vi "Set and get merit factor array.vi"(7 "action":enum16{"set", "get", "initialise"}(ring)=enum."initialise", 8 "error in (no error)":errorcluster, 9 "array size":i32=5, 10 "merit factor":dbl, 11 "RSA in":refnum<class "RSA.lvclass">) -> (0 "error out":errorcluster, 1 "current merit factor":dbl, 2 "merit factor array":dbl[](array[numeric]), 3 "RSA out":refnum<class "RSA.lvclass">)   [LabVIEW 2012, in "RSA.lvclass"]
uses:
  RSA.lvclass
  RSA.lvclass/RSA.ctl
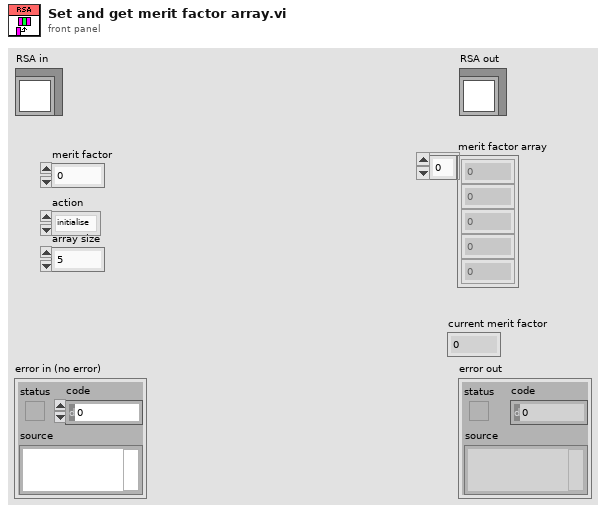
[diagram p1: front panel]
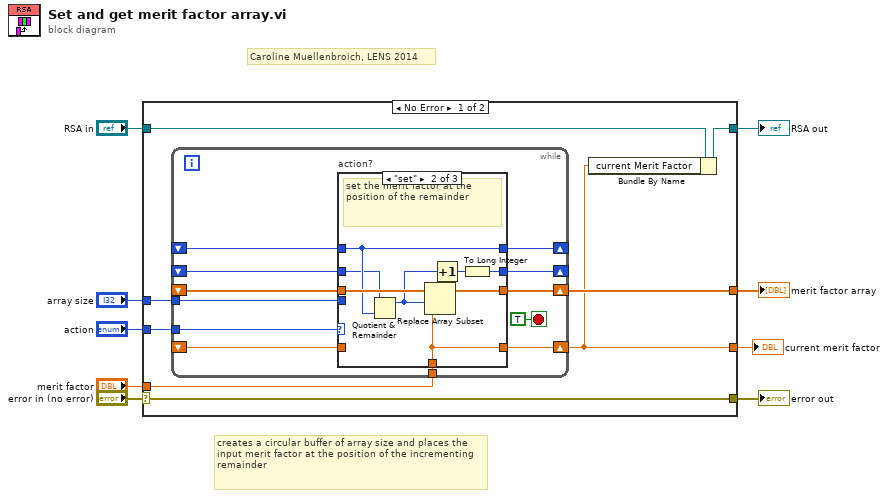
[diagram p0: block diagram]
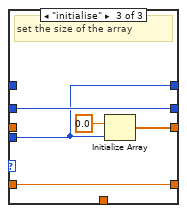
[diagram p3: hidden frame]
diagram:
  # "creates a circular buffer of array size and places the input merit factor at the position of the incrementing remainder"
  # "Caroline Muellenbroich, LENS 2014"
  n1 = case shown="No Error" "error in (no error)" {
    selector: "error in (no error)" -> [w17 w48]
    tunnel: [w17 w48] -> w8
    tunnel: [w11 w47] -> w6
    tunnel: "RSA in" -> [w12 w47]
    tunnel: "merit factor" -> [w13 _]
    tunnel: "action" -> [w16 _]
    tunnel: [w15 _] -> w3
    tunnel: "array size" -> [w14 _]
    tunnel: [w10 _] -> w1
    frame No Error {
      n2 = while {
        shift-right: [w27] -> w15
        shift-left: _ -> [w24]
        shift-right: [w26] -> _
        shift-left: _ -> [w25]
        tunnel: w16 -> [w23]
        shift-right: [w21] -> _
        shift-left: _ -> [w22]
        tunnel: w14 -> [w20]
        shift-right: [w19] -> w10
        shift-left: _ -> [w28]
        tunnel: w13 -> [w18]
        stop <- TRUE stop-if-true
        n3 = case "action?" shown="\"set\"" w23 {
          tunnel: w28 -> [w30 _ w42]
          tunnel: [w32 w39 w43] -> w27
          tunnel: [w33 w38 w46] -> w26
          tunnel: w25 -> [w33 w35 w46]
          tunnel: w24 -> [w32 w40 _]
          tunnel: w22 -> [w31 w37 _]
          tunnel: [w31 w37 w44] -> w21
          tunnel: w20 -> [_ _ w44]
          tunnel: [w30 w36 w42] -> w19
          tunnel: w18 -> [_ w36 _]
          frame "get", Default {
            # "get the array"
          }
          frame "set" {
            # "set the merit factor at the position of the remainder"
            n4 = Quotient & Remainder(x=w35, y=w37) -> (x-y*floor(x/y)=w34:i32)  [unwired: 1 out]
            n5 = Replace Array Subset(array=w40, new element=w36, index=w34) -> (w39:dbl[])
            n6 = Increment(x=w34) -> (x+1=w41:i32)
            n7 = To Long Integer(number=w41) -> (32bit integer=w38:i32)
          }
          frame "initialise" {
            # "set the size of the array"
            n8 = Initialize Array(0.0 ("merit factor"), w44) -> (w43:dbl[])
          }
        }
      }
      n9 = Bundle By Name(cluster=w12, "current Merit Factor"=w10) -> (w11:refnum<class "RSA.lvclass">)
    }
    frame Error {
    }
  }
  "error out" <- w8
  "RSA out" <- w6
  "merit factor array" <- w3
  "current merit factor" <- w1
